vi "Launcher.vi"(11 "Button 1":bool) -> ()   [LabVIEW 2012]
panel:
  in  "button clicks":dbl
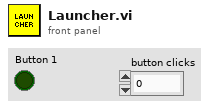
[diagram p1: front panel]
types:
  T1 = typedef "WPI_MotorControlDeviceRef.ctl" = cluster{"DeviceStatus":errorcluster, "Type":enum16{"PWM", "CAN"}, "PWM":cluster{"Digital Module":T2, "PWM Channel":T3, "DeadBand":T4}, "CAN":cluster{"Device Number":u8, "Control Mode":T5, "Semaphore":T6, "Max Vout":dbl}, "Invert":bool, "TransformRef":T7, "InvTransformRef":T7}
  T2 = typedef "FPGA_TypedefDigitalModule.ctl" = enum16{"Digital Module 1", "Digital Module 2"}
  T3 = typedef "FPGA_DIOPWMChannel.ctl" = enum8{"PWM 1", "PWM 2", "PWM 3", "PWM 4", "PWM 5", "PWM 6", "PWM 7", "PWM 8", "PWM 9", "PWM 10", "Invalid"}
  T4 = typedef "WPI_PWMDeadband.ctl" = cluster{"Name":string, "maxPositivePwm":i32, "minPositivePwm":i32, "centerPwm":i32, "maxNegativePwm":i32, "minNegativePwm":i32, "angularRange":u16}
  T5 = typedef "WPI_CANJaguar_ControlMode.ctl" = enum8{"Percent VBus", "Current", "Speed", "Position", "Voltage"}
  T6 = typedef "Semaphore RefNum" = refnum<k1>
  T7 = typedef "WPI_PWMTransform_ConPane.ctl" = refnum<vi>
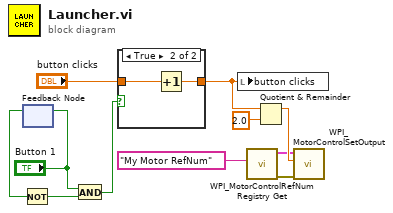
[diagram p0: block diagram]
diagram:
  n1 = feedback-in #1("Button 1") -> ()
  n2 = feedback #1() -> (w11:bool)  [unwired: 1 in]
  n3 = Not(x=w11) -> (.not. x?=w10:bool)
  n4 = And(x="Button 1", y=w10) -> (x .and. y?=w8:bool)
  n5 = case shown="True" w8 {
    tunnel: "button clicks" -> [w12 w14]
    tunnel: [w12 w13] -> w6
    frame False {
    }
    frame True {
      n6 = Increment(x=w14) -> (x+1=w13:dbl)
    }
  }
  n7 = local write "button clicks"(w6) -> ()
  n8 = call <vilib>:"WPI_MotorControlRefNum Registry Get.vi"("refnum name"="My Motor RefNum") -> ("error out"=w3:errorcluster, "MotorControlDevRef"=w1:T1)  [unwired: 9 in]
  n9 = Quotient & Remainder(x=w6, y=2.0) -> (x-y*floor(x/y)=w2:dbl)  [unwired: 1 out]
  n10 = call <vilib>:"WPI_MotorControlSetOutput.vi"("error in (no error)"=w3, "Output"=w2, "MotorControlDevRef"=w1) -> ()  [unwired: 6 in, 3 out]
